vi "ManualOverrideOCU.vi"() -> ()   [LabVIEW 2011]
uses:
  2-RIO/2 Typedefs/manual override.ctl
  2-RIO/2 Typedefs/setpoints to boat.ctl
  2-RIO/2 Typedefs/sail setpt.ctl
  2-RIO/2 Typedefs/rudder angle.ctl
  <vilib>/Utility/inputDevices.llb/closeKeyboard.vi
  2-RIO/2 Globals/2 Global.vi
  <vilib>/Utility/inputDevices.llb/keyboardAcquire.vi
panel:
  out "Manual Override Cluster":T1
  in  "OVERRIDE?":bool
  out "keys pressed":T5(array[ring])
  out "Rudder":u8
  out "Sails":u8
  in  "VI stop":bool
  in  "Full Port":bool
  in  "Port":bool
  in  "Full Starboard":bool
  in  "Starboard":bool
  out "Sent PWM Rudder Value":u8(slide) scale=250.0..50.0
  out "Sent PWM Sail Value":u8(slide) scale=250.0..50.0
  in  "Full In":bool
  in  "Sheet In":bool
  in  "Full Out":bool
  in  "Sheet Out":bool
  # "This is the Manual Override OCU:\nMake a manual override interface that can be added to the OCU (complete with keyboard control), and a typedef for the data the interface outputs. Make a separate VI that inputs data with this typedef and uses it to actually control the small RC boat. Use the system diagram (in 'required documentation' below) for reference.\nCommit code to the appropriate folders on the SVN repository."
  # "SAIL CONTROL"
  # "OUT = 90"
  # "UP"
  # "IN = 210"
  # "DOWN"
  # "RUDDER CONTROL"
  # "PORT = 210"
  # "STARB = 90"
  # "LEFT"
  # "RIGHT"
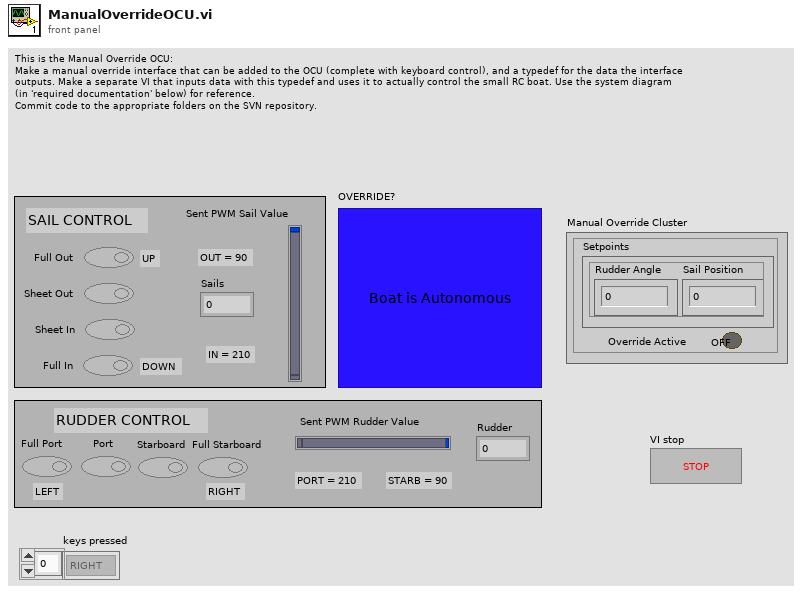
[diagram p1: front panel]
types:
  T1 = typedef "manual override.ctl" = cluster{"Override Active":bool, "Setpoints":T2}
  T2 = typedef "setpoints to boat.ctl" = cluster{"Sail Position":T3, "Rudder Angle":T4}
  T3 = typedef "sail setpt.ctl" = dbl
  T4 = typedef "rudder angle.ctl" = dbl
  T5 = enum16{"0", "1", "2", "3", "4", "5", "6", "7", "8", "9", "A", "B", "C", "D", "E", "F", "G", "H", "I", "J", "K", "L", "M", "N", "O", "P", "Q", "R", "S", "T", "U", "V", "W", "X", "Y", "Z", "F1", "F2", "F3", "F4", "F5", "F6", "F7", "F8", "F9", "F10", "F11", "F12", "F13", "F14", "F15", "ADD", "BACK", "BACKSLASH", "CAPITAL", "COMMA", "DECIMAL", "DELETE", "DIVIDE", "DOWN", "END", "EQUALS", "ESCAPE", "GRAVE (`)", "HOME", "INSERT", "LBRACKET", "LCONTROL", "LEFT", "L ALT", "LSHIFT", "LWIN", "MINUS", "MULTIPLY", "NEXT", "NUMLOCK", "NUMPAD_0", "NUMPAD_1", "NUMPAD_2", "NUMPAD_3", "NUMPAD_4", "NUMPAD_5", "NUMPAD_6", "NUMPAD_7", "NUMPAD_8", "NUMPAD_9", "PAUSE", "PERIOD", "PRIOR (PG UP)", "RBRACKET", "RCONTROL", "RETURN", "RIGHT", "R ALT", "RSHIFT", "RWIN", "SCROLL", "SEMICOLON", "SLASH", "SPACE", "SUBTRACT", "TAB", "UP", "ENTER (num pad)", "' (quote)"}[]
  T6 = enum16{"0", "1", "2", "3", "4", "5", "6", "7", "8", "9", "A", "B", "C", "D", "E", "F", "G", "H", "I", "J", "K", "L", "M", "N", "O", "P", "Q", "R", "S", "T", "U", "V", "W", "X", "Y", "Z", "F1", "F2", "F3", "F4", "F5", "F6", "F7", "F8", "F9", "F10", "F11", "F12", "F13", "F14", "F15", "ADD", "BACK", "BACKSLASH", "CAPITAL", "COMMA", "DECIMAL", "DELETE", "DIVIDE", "DOWN", "END", "EQUALS", "ESCAPE", "GRAVE (`)", "HOME", "INSERT", "LBRACKET", "LCONTROL", "LEFT", "L ALT", "LSHIFT", "LWIN", "MINUS", "MULTIPLY", "NEXT", "NUMLOCK", "NUMPAD_0", "NUMPAD_1", "NUMPAD_2", "NUMPAD_3", "NUMPAD_4", "NUMPAD_5", "NUMPAD_6", "NUMPAD_7", "NUMPAD_8", "NUMPAD_9", "PAUSE", "PERIOD", "PRIOR (PG UP)", "RBRACKET", "RCONTROL", "RETURN", "RIGHT", "R ALT", "RSHIFT", "RWIN", "SCROLL", "SEMICOLON", "SLASH", "SPACE", "SUBTRACT", "TAB", "UP", "ENTER (num pad)", "' (quote)"}
  T7 = cluster{"OVERRIDE?":bool, cluster{"element":u8, "element":u8}}
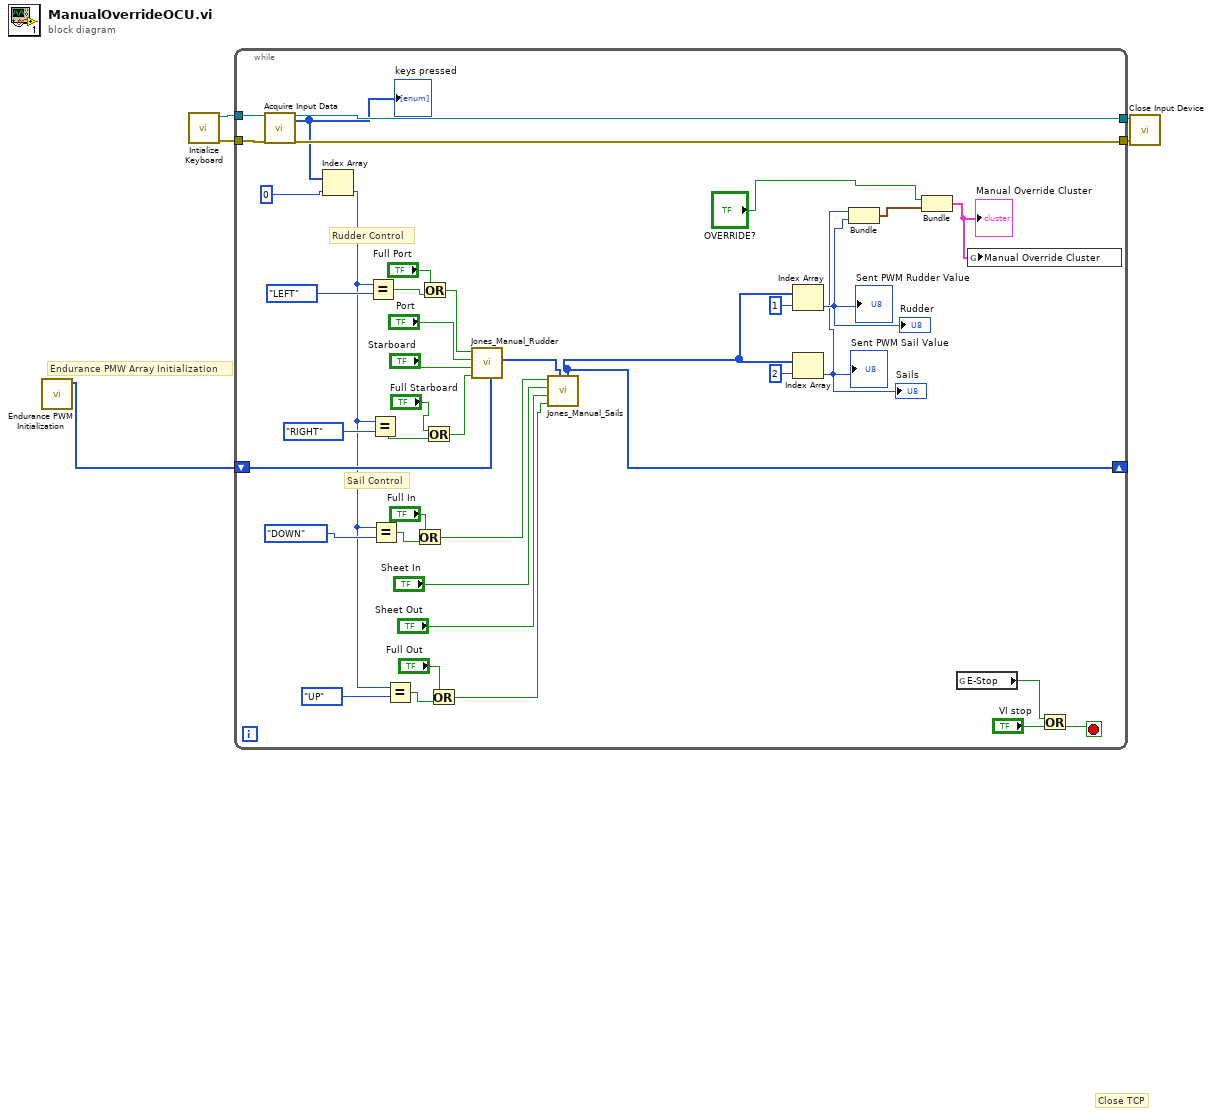
[diagram p0: block diagram]
diagram:
  # "Endurance PMW Array Initialization"
  # "Close TCP"
  n1 = call "Endurance PWM Initialization.vi"() -> ("Array"=w5:u8[])  [unwired: 11 in]
  n2 = call <vilib>:"Intialize Keyboard.vi"() -> ("error out"=w4:errorcluster, "device ID"=w3:refnum<k1>)  [unwired: 10 in]
  n3 = while {
    shift-right: [w13] -> _
    shift-left: w5 -> [w34]
    tunnel: w4 -> [w42]
    tunnel: w3 -> [w41]
    tunnel: [w40] -> w2
    tunnel: [w39] -> w1
    stop <- w7 stop-if-true
    # "Sail Control"
    # "Rudder Control"
    n4 = call-poly <vilib>:"Acquire Input Data.vi"("device ID"=w41, "error in (no error)"=w42) -> ("device ID"=w40:refnum<k1>, "keys pressed"=w38:T5, "error out"=w39:errorcluster)  [unwired: 15 in]
    "keys pressed" <- w38
    n5 = Index Array(array=w38, index=0) -> (element=w18:T6)
    n6 = Equal?(x=w18, y=T6."LEFT" ("element 2")) -> (x = y?=w29:bool)
    n7 = Equal?(x=w18, y=T6."RIGHT" ("element 2")) -> (x = y?=w24:bool)
    n8 = Equal?(x=w18, y=T6."DOWN" ("element 2")) -> (x = y?=w21:bool)
    n9 = Equal?(x=w18, y=T6."UP" ("element 2")) -> (x = y?=w16:bool)
    n10 = Or(x="Full In", y=w21) -> (x .or. y?=w20:bool)
    n11 = Or(x="Full Port", y=w29) -> (x .or. y?=w27:bool)
    n12 = Or(x="Full Starboard", y=w24) -> (x .or. y?=w25:bool)
    n13 = Or(x="Full Out", y=w16) -> (x .or. y?=w14:bool)
    n14 = call "Jones_Manual_Rudder.vi"("Full Port"=w27, "Port"="Port", "Starboard"="Starboard", "Full Starboard"=w25, "Array"=w34) -> ("Array 2"=w31:u8[])  [unwired: 3 in]
    n15 = call "Jones_Manual_Sails.vi"("Full In"=w20, "Sheet In"="Sheet In", "Sheet Out"="Sheet Out", "Full Out"=w14, "Array"=w31) -> ("Array 2"=w13:u8[])  [unwired: 5 in]
    n16 = Index Array(array=w13, index=1) -> (element=w12:u8)
    "Sent PWM Rudder Value" <- w12
    "Rudder" <- w12
    n17 = Index Array(array=w13, index=2) -> (element=w11:u8)
    "Sent PWM Sail Value" <- w11
    "Sails" <- w11
    n18 = Bundle("element"=w11, "element"=w12) -> (w10:cluster{"element":u8, "element":u8})  [unwired: 1 in]
    n19 = Bundle("OVERRIDE?"="OVERRIDE?", w10) -> (w8:T7)  [unwired: 1 in]
    "Manual Override Cluster" <- w8
    n20 = global read "2 Global.vi" "E-Stop"() -> (w6:bool)
    n21 = global write "2 Global.vi" "Manual Override Cluster"(w8) -> ()
    n22 = Or(x=w6, y="VI stop") -> (x .or. y?=w7:bool)
  }
  n23 = call-poly <vilib>:"Close Input Device.vi"("error in (no error)"=w1, "device ID"=w2) -> ()  [unwired: 8 in, 1 out]
